vi "GFITS_VAR_Hdrs.vi"(0 "action":enum16{"read", "write"}(ring), 1 "nkeys before in":i32[](array[numeric]), 2 "nkeys after in":i32[](array[numeric]), 5 "GFITS_allkeys in":string[][][](array[string]), 7 "GFITS_beforein":string[][][](array[string]), 9 "GFITS_after in":string[][][](array[string]), 11 "geom info in":bool) -> (6 "GFITS_allkeys":string[][][](array[string]), 8 "GFITS_before":string[][][](array[string]), 10 "GFITS_after":string[][][](array[string]), 12 "nkeys before":i32[](array[numeric]), 13 "nkeys after":i32[](array[numeric]), 15 "geom info":bool)   [LabVIEW 2016]
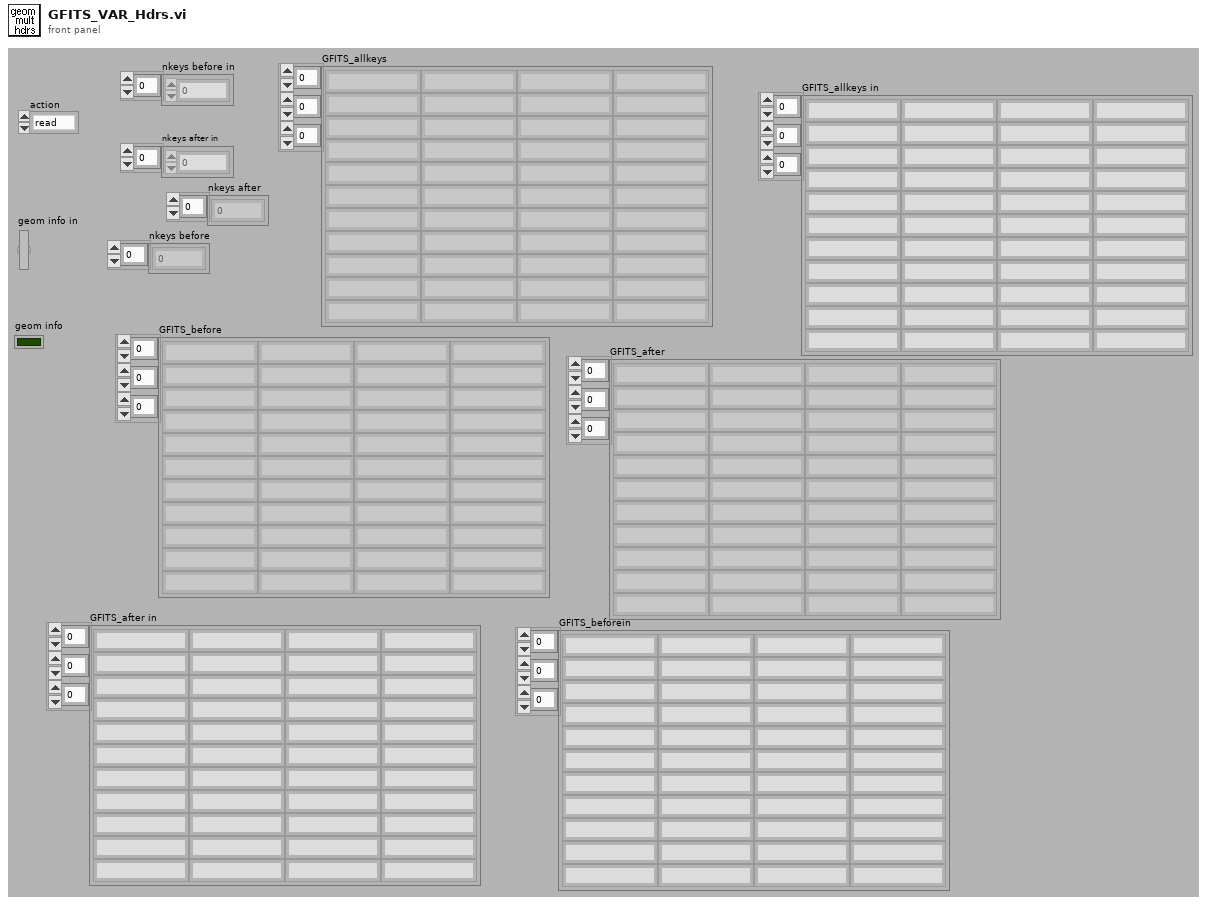
[diagram p1: front panel]
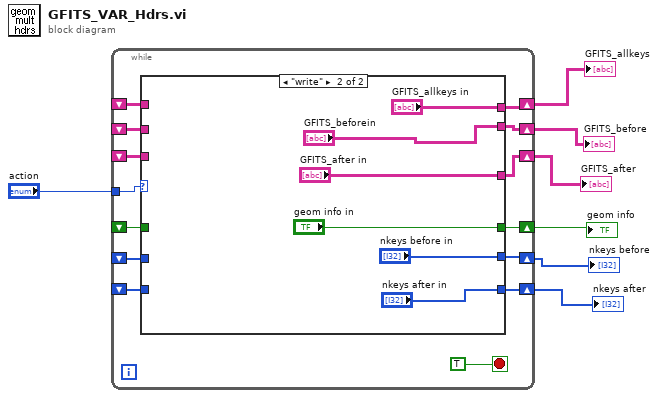
[diagram p0: block diagram]
diagram:
  n1 = while {
    tunnel: "action" -> [w20]
    shift-right: [w18] -> w4
    shift-left: _ -> [w19]
    shift-right: [w17] -> w3
    shift-left: _ -> [w14]
    shift-right: [w16] -> w6
    shift-left: _ -> [w13]
    shift-right: [w15] -> w5
    shift-left: _ -> [w12]
    shift-right: [w11] -> w2
    shift-left: _ -> [w9]
    shift-right: [w10] -> w1
    shift-left: _ -> [w8]
    stop <- TRUE stop-if-true
    n2 = case shown="\"write\"" w20 {
      tunnel: w19 -> [w27 _]
      tunnel: [w27 "GFITS_allkeys in"] -> w18
      tunnel: [w26 "GFITS_beforein"] -> w17
      tunnel: [w25 "GFITS_after in"] -> w16
      tunnel: [w24 "geom info in"] -> w15
      tunnel: w14 -> [w26 _]
      tunnel: w13 -> [w25 _]
      tunnel: w12 -> [w24 _]
      tunnel: [w23 "nkeys before in"] -> w11
      tunnel: [w22 "nkeys after in"] -> w10
      tunnel: w9 -> [w23 _]
      tunnel: w8 -> [w22 _]
      frame "read", Default {
      }
      frame "write" {
      }
    }
  }
  "GFITS_allkeys" <- w4
  "GFITS_before" <- w3
  "GFITS_after" <- w6
  "geom info" <- w5
  "nkeys after" <- w1
  "nkeys before" <- w2
